vi "Format Word for CSV.vi"(10 "data word format":T1="Hexadecimal", 11 "word":T2) -> (3 "string array":string[](array[string]))   [LabVIEW 2020, in "AIM ARINC 429 Engine.lvlib" / "Implementation.lvlib" / "CSV Word Logger.lvclass"]
uses:
  CSV Word Logger.lvclass
  Word.ctl
  Implementation.lvlib
  Shared/Data Word Format.ctl
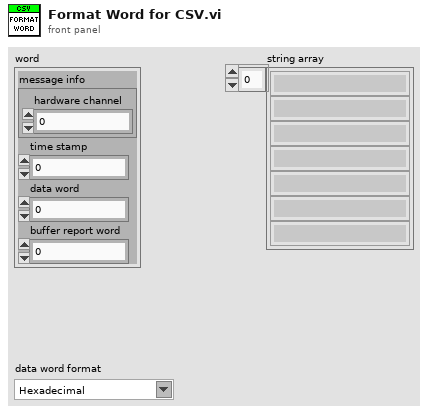
[diagram p1: front panel]
types:
  T1 = typedef "Data Word Format.ctl" = string
  T2 = typedef "AIM ARINC 429 Engine.lvlib/Implementation.lvlib/Word.ctl" = cluster{"message info":cluster{"hardware channel":u8}, "time stamp":dbl, "data word":u32, "buffer report word":u32}
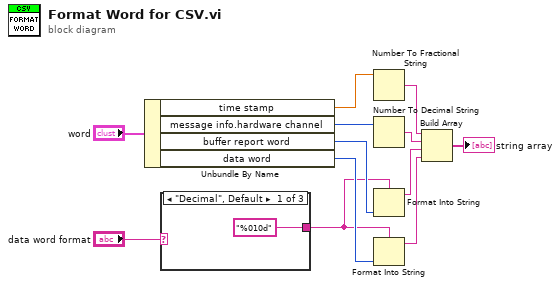
[diagram p0: block diagram]
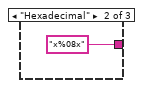
[diagram p2: hidden frame]
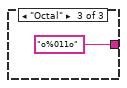
[diagram p3: hidden frame]
diagram:
  n1 = Unbundle By Name("word") -> ("time stamp"=w7:dbl, "message info.hardware channel"=w6:u8, "buffer report word"=w3:u32, "data word"=w11:u32)
  n2 = case shown="\"Decimal\", Default" "data word format" {
    tunnel: ["%010d" ("format string") "x%08x" ("format string") "o%011o" ("format string")] -> w1
    frame "Decimal", Default {
    }
    frame "Hexadecimal" {
    }
    frame "Octal" {
    }
  }
  n3 = Number To Fractional String(number=w7) -> (F-format string=w9:string)  [unwired: 3 in]
  n4 = Number To Decimal String(number=w6) -> (decimal integer string=w8:string)  [unwired: 1 in]
  n5 = Format Into String(format string=w1, w3) -> (resulting string=w2:string)  [unwired: 2 in, 1 out]
  n6 = Format Into String(format string=w1, w11) -> (resulting string=w12:string)  [unwired: 2 in, 1 out]
  n7 = Build Array(w9, w8, w2, w12) -> (→"string array":string[])
